vi "bit val unsigned 8.vi"(9 "bit num":i8, 10 "x":u8) -> (2 "BV":bool)   [LabVIEW 2010]
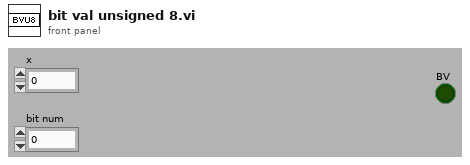
[diagram p1: front panel]
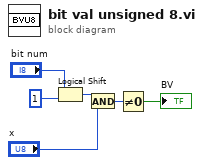
[diagram p0: block diagram]
diagram:
  n1 = Logical Shift(y="bit num", x=u8 1) -> (x << y=w4:u8)
  n2 = And(x=w4, y="x") -> (x .and. y?=w2:u8)
  n3 = Not Equal To 0?(x=w2) -> (x != 0?=→"BV":bool)
